vi "23_1c.vi"() -> ()   [LabVIEW 2020]
uses:
  <vilib>/Analysis/1siggen.llb/Ramp Pattern by Delta.vi
  <vilib>/Analysis/NI_AALBase.lvlib
panel:
  out "Array":u64[](array[numeric])=[6, 9, 8, 5, 2, 4, 3, 7, 1]
  in  "Moves":i32=100
  in  "Cups":dbl=9.0 format="%#_13g"
  in  "Switch":bool
  in  "Input":string="925176834"
  in  "Input Test":string="389125467"
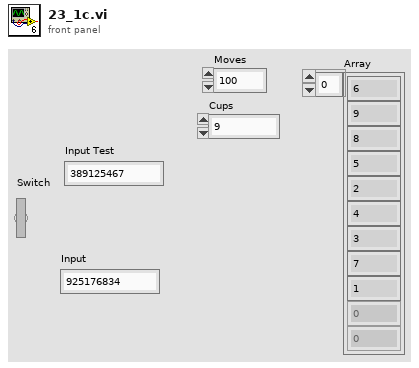
[diagram p1: front panel]
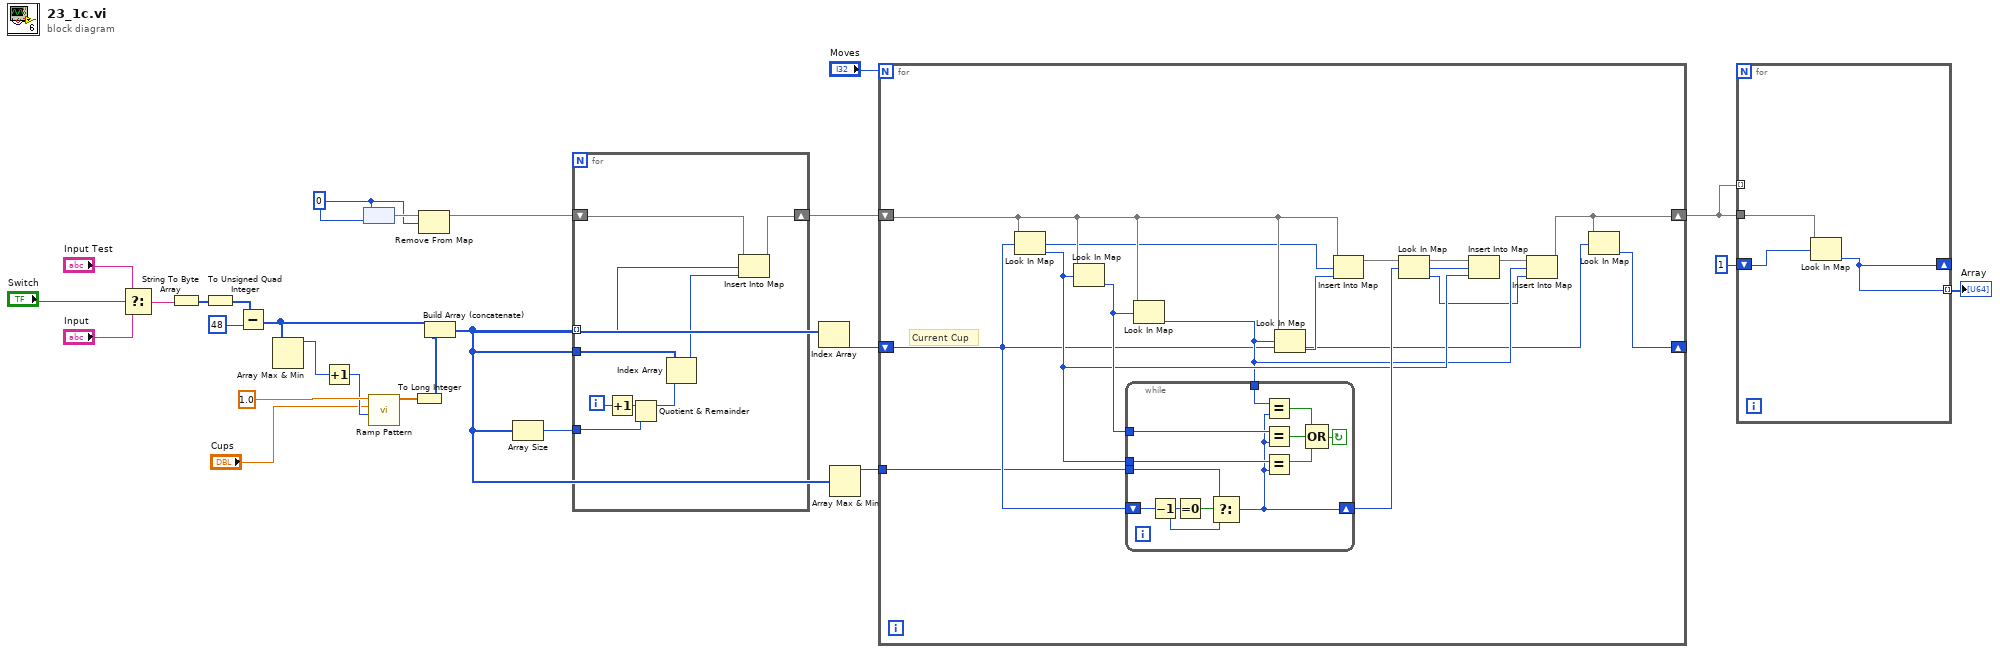
[diagram p0: block diagram]
diagram:
  w11 = u64 0
  n1 = Select(t="Input Test", s="Switch", f="Input") -> (s? t:f=w23:string)
  n2 = String To Byte Array(string=w23) -> (unsigned byte array=w22:u8[])
  n3 = To Unsigned Quad Integer(1:w22) -> (0:w20:u64[])
  n4 = Subtract(x=w20, y=u64 48) -> (x-y=w14:u64[])
  n5 = Array Max & Min(array=w14) -> (max value=w16:u64)  [unwired: 3 out]
  n6 = Increment(x=w16) -> (x+1=w17:u64)
  n7 = node(w11, w11) -> (w12:map{u64, u64})
  n8 = call-poly <vilib>:"Ramp Pattern.vi"("start"=w17, "end"="Cups", "delta"=1.0) -> ("Ramp Pattern"=w18:dbl[])  [unwired: 6 in, 2 out]
  n9 = To Long Integer(number=w18) -> (32bit integer=w13:i32[])
  n10 = Remove From Map(10:w11, 11:w12) -> (3:w10:map{u64, u64})  [unwired: 2 out]
  n11 = Build Array (concatenate)(w14, w13) -> (w6:u64[])
  n12 = Array Size(array=w6) -> (size(s)=w9:i32)
  n13 = for {
    shift-right: [w30] -> w8
    shift-left: w10 -> [w32]
    tunnel: w6 -> [w31] mode=indexing
    tunnel: w6 -> [w29]
    tunnel: w9 -> [w33]
    i -> [w35]
    n14 = Increment(x=w35) -> (x+1=w34:i32)
    n15 = Quotient & Remainder(x=w34, y=w33) -> (x-y*floor(x/y)=w28:i32)  [unwired: 1 out]
    n16 = Index Array(array=w29, index=w28) -> (element=w27:u64)
    n17 = Insert Into Map(map in=w32, key=w31, value=w27) -> (map out=w30:map{u64, u64})  [unwired: 2 out]
  }
  n18 = Index Array(array=w6) -> (element=w7:u64)  [unwired: 1 in]
  n19 = Array Max & Min(array=w6) -> (max value=w5:u64)  [unwired: 3 out]
  n20 = for {
    N: "Moves" -> [_]
    shift-right: [w39] -> w2
    shift-left: w8 -> [w48]
    shift-right: [w37] -> _
    shift-left: w7 -> [w38]
    tunnel: w5 -> [w36]
    # "Current Cup"
    n21 = Look In Map(map=w48, key=w38) -> (value=w43:u64)  [unwired: 1 in, 1 out]
    n22 = Look In Map(map=w48, key=w43) -> (value=w46:u64)  [unwired: 1 in, 1 out]
    n23 = Look In Map(map=w48, key=w46) -> (value=w41:u64)  [unwired: 1 in, 1 out]
    n24 = while {
      tunnel: w41 -> [w59]
      tunnel: w46 -> [w58]
      tunnel: w43 -> [w57]
      shift-right: [w52] -> w44
      shift-left: w38 -> [w60]
      tunnel: w36 -> [w49]
      stop <- w53 continue-if-true
      n25 = Decrement(x=w60) -> (x-1=w50:u64)
      n26 = Equal To 0?(x=w50) -> (x = 0?=w51:bool)
      n27 = Select(t=w49, s=w51, f=w50) -> (s? t:f=w52:u64)
      n28 = Equal?(x=w59, y=w52) -> (x = y?=w55:bool)
      n29 = Equal?(x=w58, y=w52) -> (x = y?=w56:bool)
      n30 = Equal?(x=w57, y=w52) -> (x = y?=w54:bool)
      n31 = Compound Arithmetic op=OR(w55, w56, w54) -> (w53:bool)
    }
    n32 = Look In Map(map=w48, key=w41) -> (value=w47:u64)  [unwired: 1 in, 1 out]
    n33 = Insert Into Map(map in=w48, key=w38, value=w47) -> (map out=w45:map{u64, u64})  [unwired: 2 out]
    n34 = Look In Map(map=w45, key=w44) -> (value=w40:u64)  [unwired: 1 in, 1 out]
    n35 = Insert Into Map(map in=w45, key=w44, value=w43) -> (map out=w42:map{u64, u64})  [unwired: 2 out]
    n36 = Insert Into Map(map in=w42, key=w41, value=w40) -> (map out=w39:map{u64, u64})  [unwired: 2 out]
    n37 = Look In Map(map=w39, key=w38) -> (value=w37:u64)  [unwired: 1 in, 1 out]
  }
  n38 = for {
    shift-right: [w63] -> _
    shift-left: u64 1 -> [w62]
    tunnel: [w63] -> w1 mode=indexing
    tunnel: w2 -> [w61]
    tunnel: w2 -> [_] mode=indexing
    n39 = Look In Map(map=w61, key=w62) -> (value=w63:u64)  [unwired: 1 in, 1 out]
  }
  "Array" <- w1
